vi "Caliper Setting UI_old.vi"(8 "error in (no error)":errorcluster, 11 "Vision_Image":T7(plugin-control)) -> (0 "error out":errorcluster, 2 "Cancel?":bool)   [LabVIEW 2015]
uses:
  Controls/CaliperType with Picture.ctl
  Controls/SelectionListEntry.ctl
  Controls/SelectionListEntryPointType.ctl
  Controls/CaliperDataEntry.ctl
  Controls/CaliperType.ctl
  Controls/CaliperResult.ctl
  Controls/Caliper_UI_Action_old.ctl
  Controls/AnalysisResultPointsAction.ctl
  Analysis/Controls/Analysis_Result_To_Caliper.ctl
panel:
  out "Result":string
  in  "DeleteCaliper":bool
  in  "CaliperList":i32(listbox)
  in  "AddCaliper":bool
  out "Result":T1
  out "CaliperEntryList":T2[](array[typedef]) {"CaliperType" items=["Distance", "Mid Point", "Perpendicular Projection", "Lines Intersection", "Angle from Horizontal", "Angle from Vertical", "Angle Defined by 3 Points", "Angle Defined by 4 Points", "Bissecting Line", "Mid Line", "Center of Mass", "Area", "Line Fit", "Circle Fit", "Ellipse Fit"]}
  out "AnalysisResultNum":i32
  out "SelectionList":T4[](array[typedef])
  out "Row":i32
  in  "Analysis Results":i32[](listbox) caption="Table"
  in  "CaliperType_w_Pic":T6 caption="Caliper Type" items=["Distance", "Mid Point", "Perpendicular Projection", "Lines Intersection", "Angle from Horizontal", "Angle from Vertical", "Angle Defined by 3 Points", "Angle Defined by 4 Points", "Bissecting Line", "Mid Line", "Center of Mass", "Area", "Line Fit", "Circle Fit", "Ellipse Fit"]
  in  "Cancel":bool
  in  "Done":bool
  in  "Run Algorithm":bool
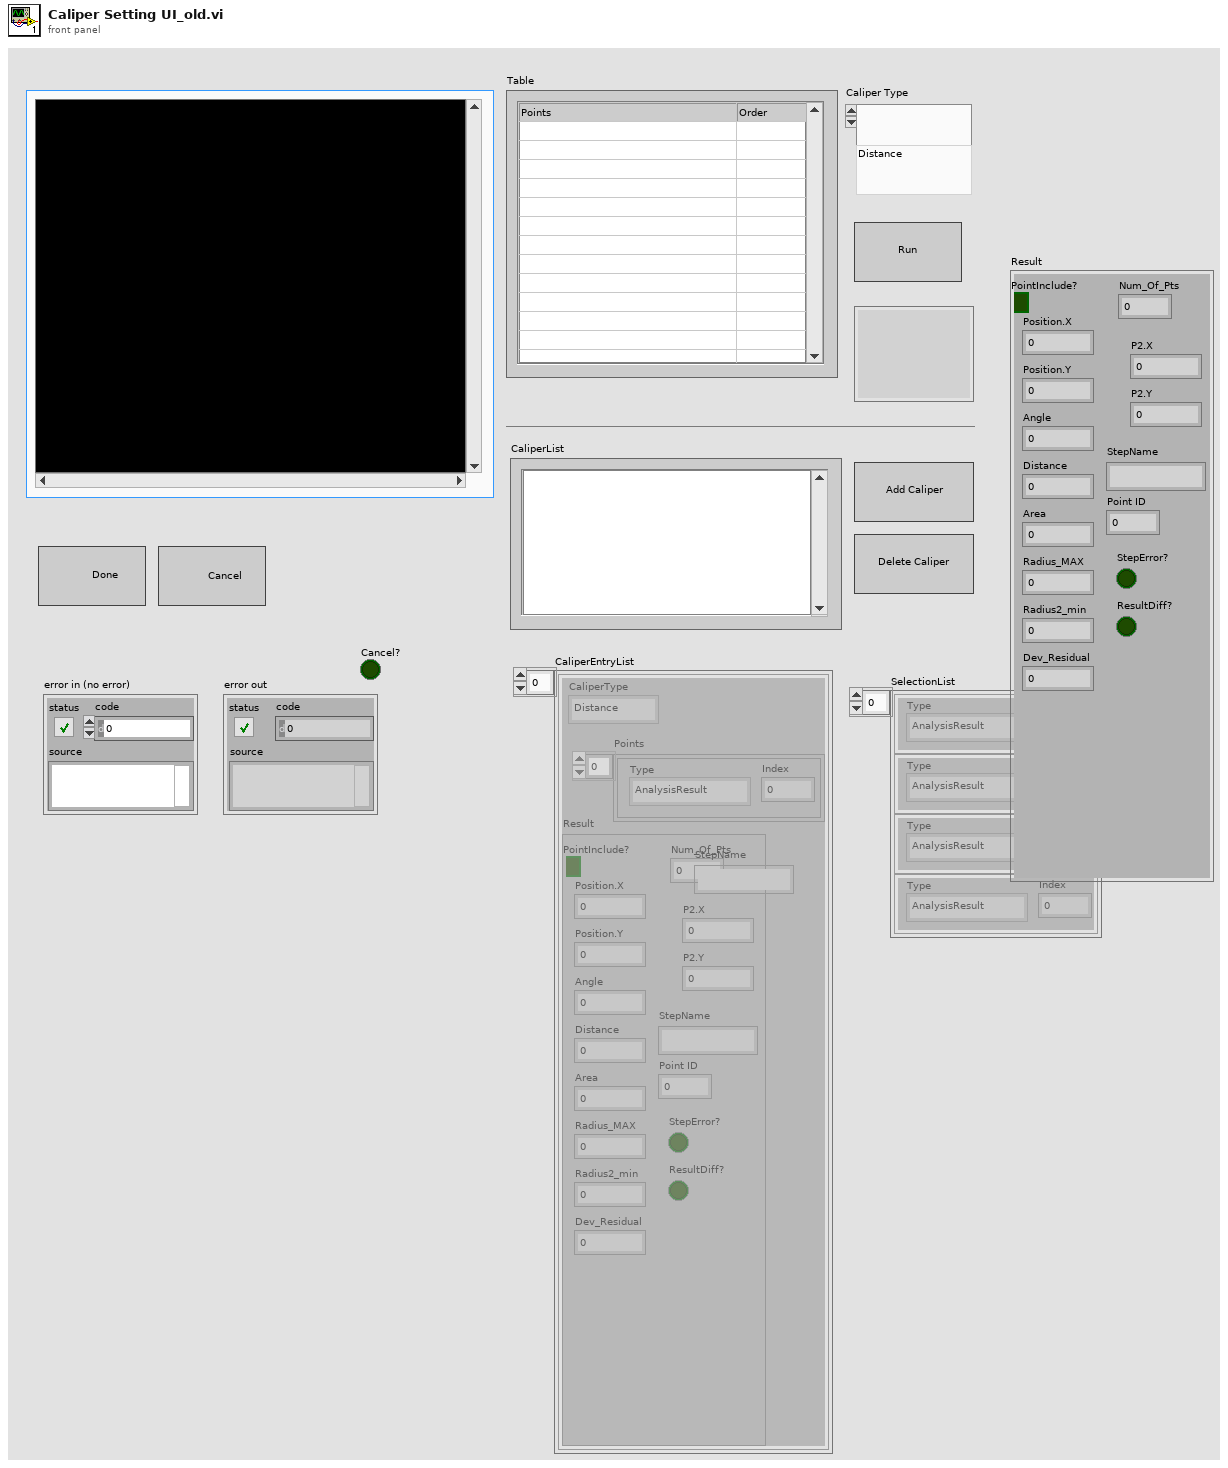
[diagram p1: front panel]
types:
  T1 = typedef "CaliperResult.ctl" = cluster{"PointInclude?":bool, "Num_Of_Pts":u8, "Position.X":dbl, "Position.Y":dbl, "Angle":dbl, "Distance":dbl, "Area":dbl, "Radius_MAX":dbl, "Radius2_min":dbl, "Dev_Residual":dbl, "P2.X":dbl, "P2.Y":dbl, "StepName":string, "Point ID":u8, "StepError?":bool, "ResultDiff?":bool}
  T2 = typedef "CaliperDataEntry.ctl" = cluster{"CaliperType":T3, "Points":T4[], "Result":T1, "StepName":string}
  T3 = typedef "CaliperType.ctl" = u32
  T4 = typedef "SelectionListEntry.ctl" = cluster{"Type":T5, "Index":i32}
  T5 = typedef "SelectionListEntryPointType.ctl" = enum16{"AnalysisResult", "CaliperResult"}
  T6 = typedef "CaliperType with Picture.ctl" = u32
  T7 = typedef "IMAQ Image.ctl" = refnum<image>
  T8 = typedef "Caliper_UI_Action_old.ctl" = enum16{"Init", "Done", "Cancel", "Run", "InitAnalysisResultTable", "UpdateSymbol", "UpdateOrderInTable", "UpdateAnalysisTable", "AddCaliperResultToTable", "AddCaliperEntry", "SetCaliperStepName", "UpdateCaliperList", "RemoveCaliperEntry", "ResetSelectionList"}
  T9 = typedef "Analysis_Result_To_Caliper.ctl" = cluster{"PointName":string, "Position_X":dbl, "Position_Y":dbl}
  T10 = typedef "AnalysisResultPointsAction.ctl" = enum16{"Init", "Add", "Delete", "ReplaceAll", "ReadAll", "Close"}
  T11 = typedef "CaliperDataEntry_SinglePoint.ctl" = cluster{"CaliperType":T3, "Points":T4[], "Result":T12, "StepName":string}
  T12 = typedef "CaliperResult_SinglePoint.ctl" = cluster{"PointInclude?":bool, "Position.X":dbl, "Position.Y":dbl, "Angle":dbl, "Distance":dbl, "Area":dbl, "Radius_MAX":dbl, "Radius2_min":dbl, "Dev_Residual":dbl, "StepName":string, "Point ID":u8, "StepError?":bool, "ResultDiff?":bool}
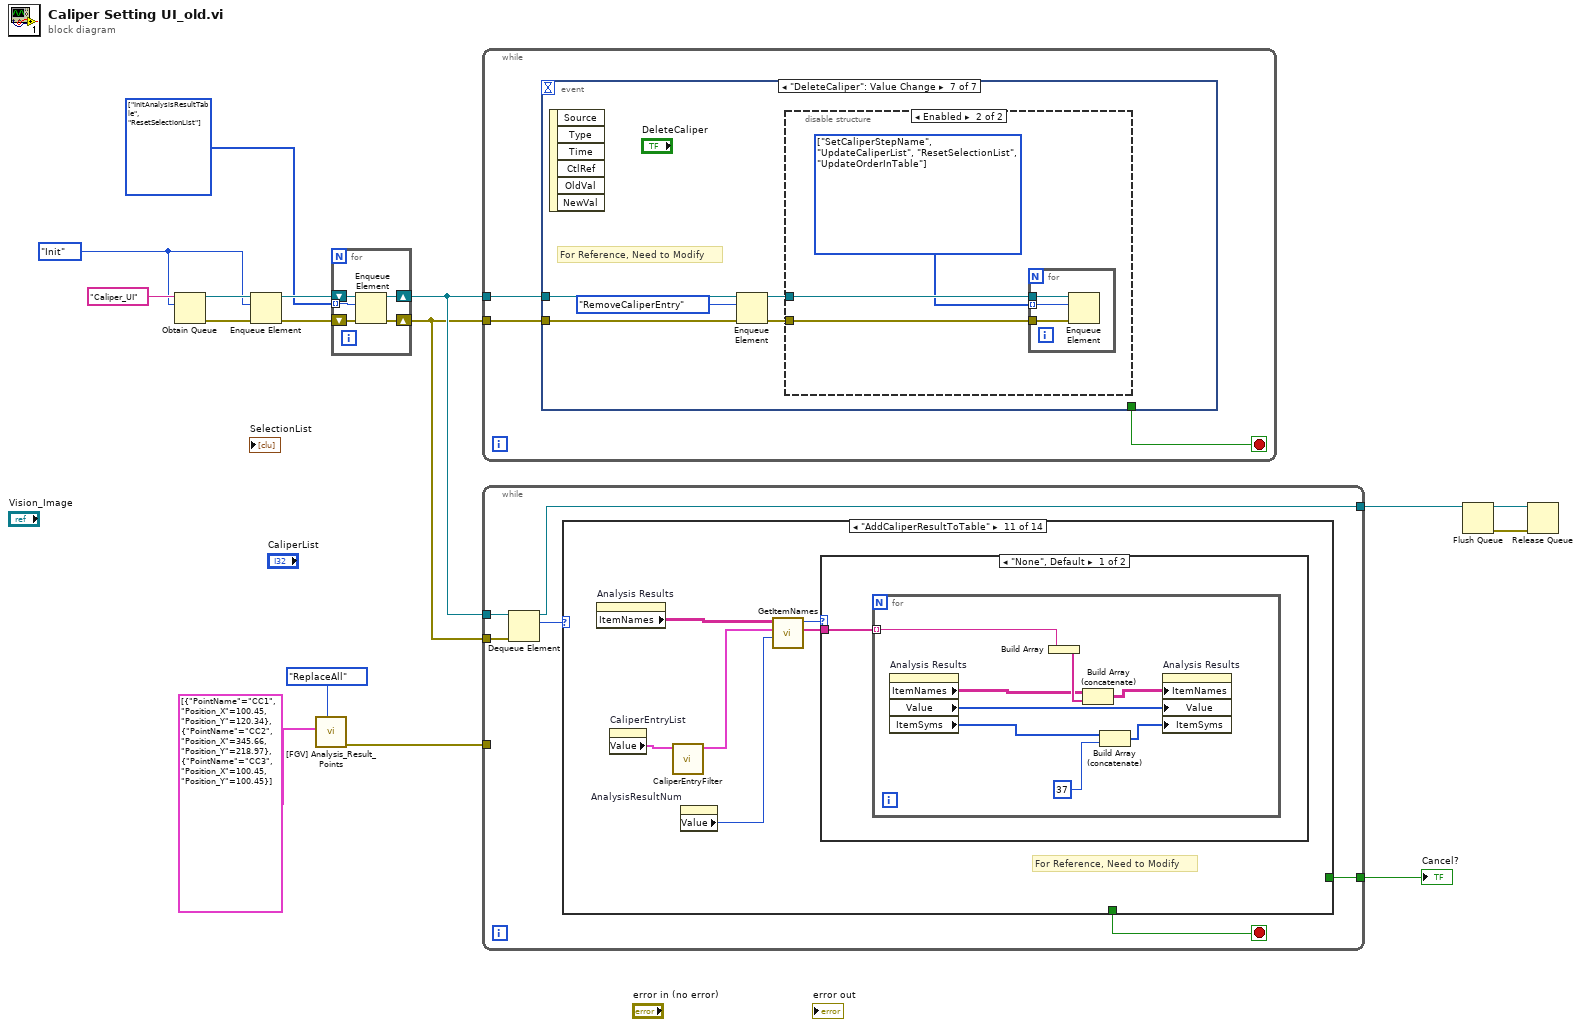
[diagram p0: block diagram]
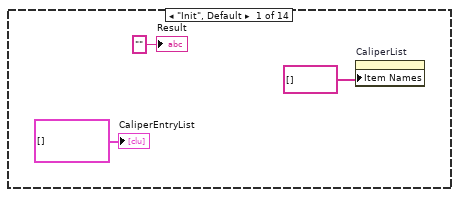
[diagram p2: hidden frame]
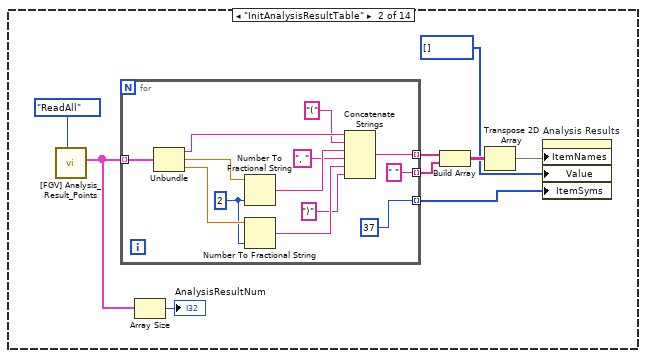
[diagram p3: hidden frame]
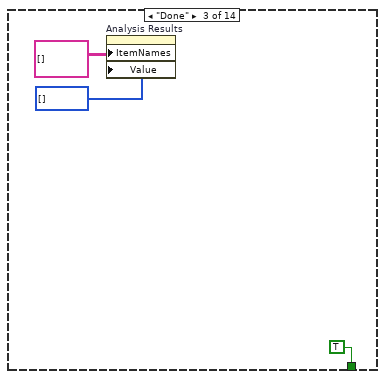
[diagram p4: hidden frame]
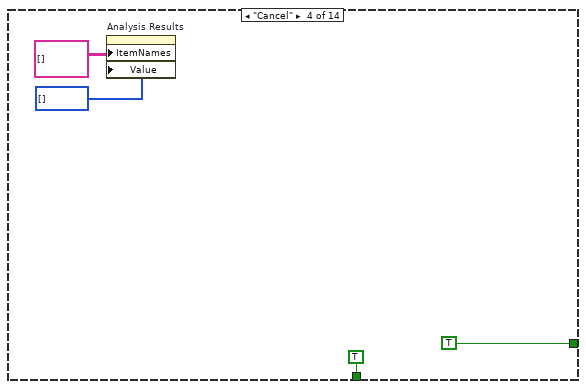
[diagram p5: hidden frame]
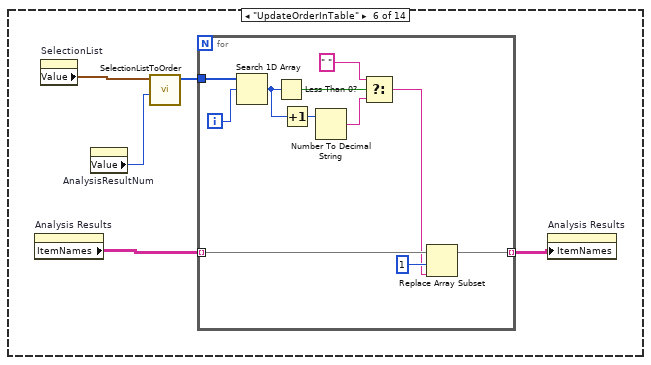
[diagram p7: hidden frame]
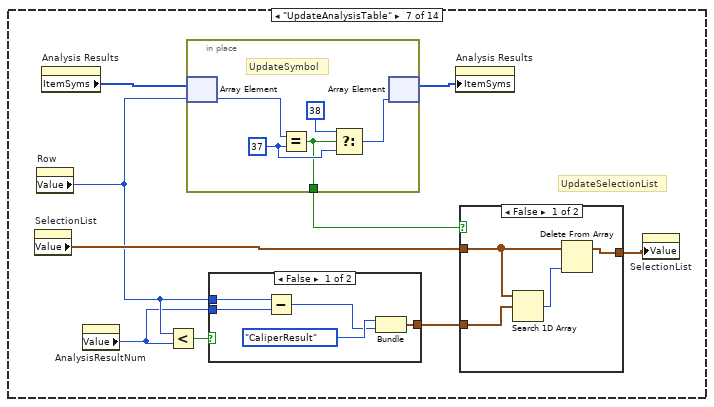
[diagram p8: hidden frame]
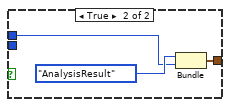
[diagram p9: hidden frame]
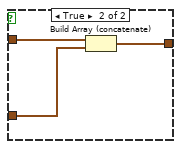
[diagram p10: hidden frame]
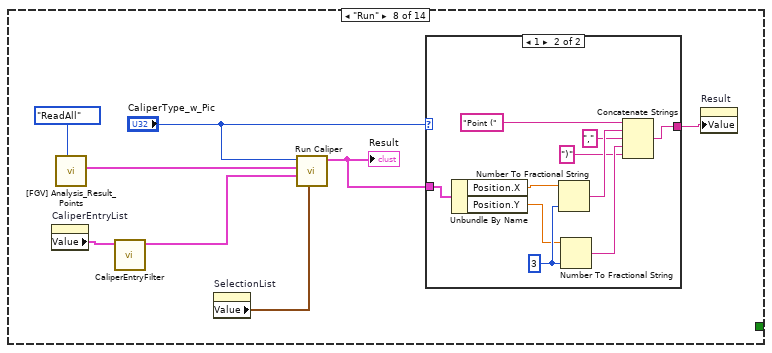
[diagram p11: hidden frame]
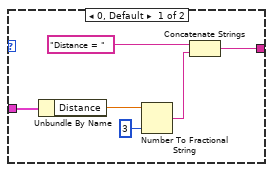
[diagram p12: hidden frame]
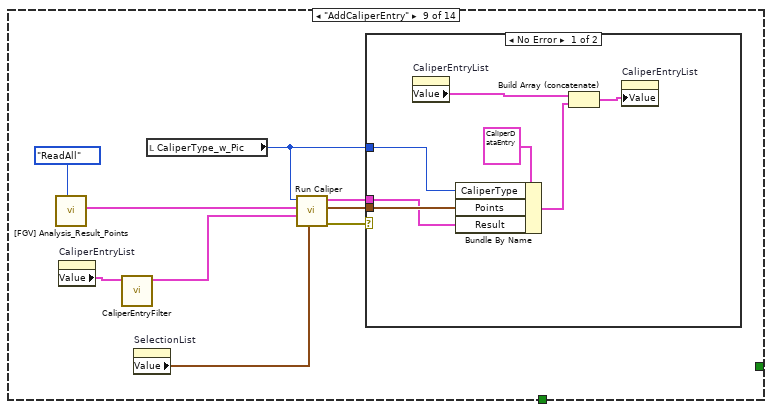
[diagram p13: hidden frame]
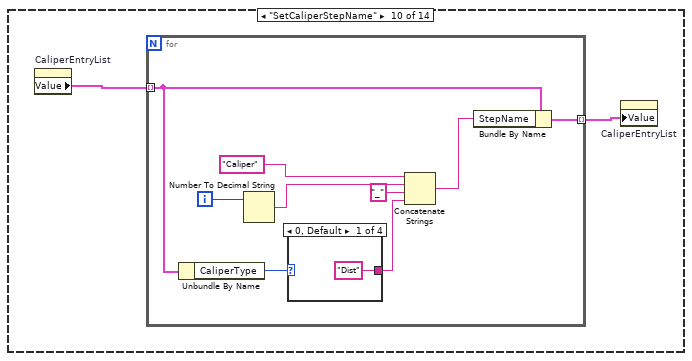
[diagram p15: hidden frame]
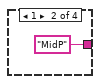
[diagram p16: hidden frame]
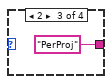
[diagram p17: hidden frame]
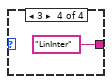
[diagram p18: hidden frame]
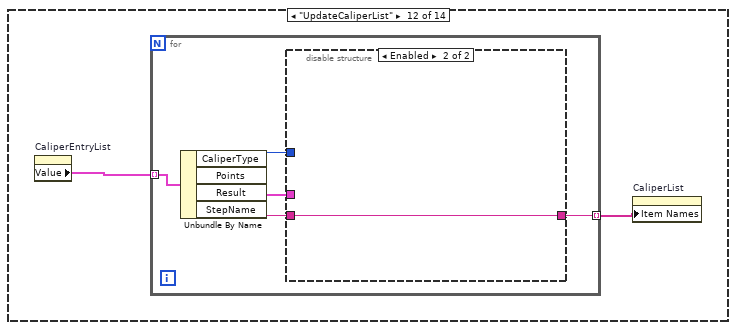
[diagram p20: hidden frame]
diagram:
  w1 = T8[] [enum."InitAnalysisResultTable", enum."ResetSelectionList"] items=["Init", "Done", "Cancel", "Run", "InitAnalysisResultTable", "UpdateSymbol", "UpdateOrderInTable", "UpdateAnalysisTable", "AddCaliperResultToTable", "AddCaliperEntry", "SetCaliperStepName", "UpdateCaliperList", "RemoveCaliperEntry", "ResetSelectionList"]
  w14 = Caliper_UI_Action_old."Init" ("CaliperAction")
  n1 = Obtain Queue(name (unnamed)="Caliper_UI", element data type=w14) -> (queue out=w15:refnum<queue>, error out=w9:errorcluster)  [unwired: 3 in, 1 out]
  n2 = Enqueue Element(queue=w15, element=w14, error in (no error)=w9) -> (queue out=w8:refnum<queue>, error out=w6:errorcluster)  [unwired: 1 in, 1 out]
  n3 = call "[FGV] Analysis_Result_Points.vi"("Action"=AnalysisResultPointsAction."ReplaceAll", "Analysis_Point_Result"=T9[] [{"PointName"="CC1", "Position_X"=100.45, "Position_Y"=120.34}, {"PointName"="CC2", "Position_X"=345.66, "Position_Y"=218.97}, {"PointName"="CC3", "Position_X"=100.45, "Position_Y"=100.45}]) -> ("error out"=w3:errorcluster)  [unwired: 8 in, 1 out]
  n4 = for {
    tunnel: w1 -> [w17] mode=indexing
    shift-right: [w20] -> w7
    shift-left: w8 -> [w21]
    shift-right: [w18] -> w5
    shift-left: w6 -> [w19]
    n5 = Enqueue Element(queue=w21, element=w17, error in (no error)=w19) -> (queue out=w20:refnum<queue>, error out=w18:errorcluster)  [unwired: 1 in, 1 out]
  }
  n6 = while {
    tunnel: w7 -> [w24]
    tunnel: w5 -> [w23]
    stop <- w22 stop-if-true
    n7 = event shown="[6] \"DeleteCaliper\": Value Change" {
      selector: _ -> [_ _ _ _ _ _ _]
      dyn-events: _ -> [_ _ _ _ _ _ _]
      timeout: _ -> [_ _ _ _ _ _ _]
      tunnel: w24 -> [_ w28 w32 w41 w45 w50 w67]
      tunnel: w23 -> [_ w27 w31 w40 w44 w49 w66]
      tunnel: [_ TRUE TRUE _ _ _ _] -> w22
      event Timeout {
        n8 = event-data() -> ()  [unwired: 1 in, 2 out]
      }
      event "Done": Value Change {
        n9 = event-data() -> ()  [unwired: 1 in, 6 out]
        n10 = Enqueue Element(queue=w28, element=Caliper_UI_Action_old."Done", error in (no error)=w27) -> ()  [unwired: 1 in, 3 out]
      }
      event "Cancel": Value Change {
        n11 = event-data() -> ()  [unwired: 1 in, 6 out]
        n12 = Enqueue Element(queue=w32, element=Caliper_UI_Action_old."Cancel", error in (no error)=w31) -> ()  [unwired: 1 in, 3 out]
      }
      event "Analysis Results": Double Click {
        n13 = event-data() -> ("Row"=→"Row":i32)  [unwired: 1 in, 8 out]
        n14 = Enqueue Element(queue=w41, element=Caliper_UI_Action_old."UpdateSymbol", error in (no error)=w40) -> (queue out=w38:refnum<queue>, error out=w37:errorcluster)  [unwired: 1 in, 1 out]
        n15 = Enqueue Element(queue=w38, element=Caliper_UI_Action_old."UpdateAnalysisTable", error in (no error)=w37) -> (queue out=w36:refnum<queue>, error out=w35:errorcluster)  [unwired: 1 in, 1 out]
        n16 = Enqueue Element(queue=w36, element=Caliper_UI_Action_old."UpdateOrderInTable", error in (no error)=w35) -> ()  [unwired: 1 in, 3 out]
      }
      event "Run Algorithm": Value Change {
        n17 = event-data() -> ()  [unwired: 1 in, 6 out]
        n18 = Enqueue Element(queue=w45, element=Caliper_UI_Action_old."Run", error in (no error)=w44) -> ()  [unwired: 1 in, 3 out]
      }
      event "AddCaliper": Value Change {
        # "For Reference, Need to Modify"
        n19 = event-data() -> ()  [unwired: 1 in, 6 out]
        n20 = Enqueue Element(queue=w50, element=Caliper_UI_Action_old."AddCaliperEntry", error in (no error)=w49) -> (queue out=w47:refnum<queue>, error out=w46:errorcluster)  [unwired: 1 in, 1 out]
        n21 = disable-structure shown="Enabled" {
          disable-tunnel: w47 -> [w55 w58]
          disable-tunnel: w46 -> [w53 w59]
          frame Disabled {
            n22 = Enqueue Element(queue=w55, element=Caliper_UI_Action_old."InitAnalysisResultTable", error in (no error)=w53) -> (queue out=w54:refnum<queue>, error out=w52:errorcluster)  [unwired: 1 in, 1 out]
            n23 = Enqueue Element(queue=w54, element=Caliper_UI_Action_old."AddCaliperResultToTable", error in (no error)=w52) -> ()  [unwired: 1 in, 3 out]
          }
          frame Enabled {
            w57 = T8[] [enum."SetCaliperStepName", enum."AddCaliperResultToTable", enum."UpdateCaliperList", enum."ResetSelectionList", enum."UpdateOrderInTable"] items=["Init", "Done", "Cancel", "Run", "InitAnalysisResultTable", "UpdateSymbol", "UpdateOrderInTable", "UpdateAnalysisTable", "AddCaliperResultToTable", "AddCaliperEntry", "SetCaliperStepName", "UpdateCaliperList", "RemoveCaliperEntry", "ResetSelectionList"]
            n24 = for {
              tunnel: w59 -> [w62]
              tunnel: w58 -> [w61]
              tunnel: w57 -> [w60] mode=indexing
              n25 = Enqueue Element(queue=w61, element=w60, error in (no error)=w62) -> ()  [unwired: 1 in, 3 out]
            }
          }
        }
      }
      event "DeleteCaliper": Value Change {
        # "For Reference, Need to Modify"
        n26 = event-data() -> ()  [unwired: 1 in, 6 out]
        n27 = Enqueue Element(queue=w67, element=Caliper_UI_Action_old."RemoveCaliperEntry", error in (no error)=w66) -> (queue out=w64:refnum<queue>, error out=w63:errorcluster)  [unwired: 1 in, 1 out]
        n28 = disable-structure shown="Enabled" {
          disable-tunnel: w64 -> [w72 w75]
          disable-tunnel: w63 -> [w70 w76]
          frame Disabled {
            n29 = Enqueue Element(queue=w72, element=Caliper_UI_Action_old."InitAnalysisResultTable", error in (no error)=w70) -> (queue out=w71:refnum<queue>, error out=w69:errorcluster)  [unwired: 1 in, 1 out]
            n30 = Enqueue Element(queue=w71, element=Caliper_UI_Action_old."AddCaliperResultToTable", error in (no error)=w69) -> ()  [unwired: 1 in, 3 out]
          }
          frame Enabled {
            w74 = T8[] [enum."SetCaliperStepName", enum."UpdateCaliperList", enum."ResetSelectionList", enum."UpdateOrderInTable"] items=["Init", "Done", "Cancel", "Run", "InitAnalysisResultTable", "UpdateSymbol", "UpdateOrderInTable", "UpdateAnalysisTable", "AddCaliperResultToTable", "AddCaliperEntry", "SetCaliperStepName", "UpdateCaliperList", "RemoveCaliperEntry", "ResetSelectionList"]
            n31 = for {
              tunnel: w76 -> [w79]
              tunnel: w75 -> [w78]
              tunnel: w74 -> [w77] mode=indexing
              n32 = Enqueue Element(queue=w78, element=w77, error in (no error)=w79) -> ()  [unwired: 1 in, 3 out]
            }
          }
        }
      }
    }
  }
  n33 = while {
    tunnel: w7 -> [w85]
    tunnel: w5 -> [w84]
    tunnel: [w82] -> w13
    tunnel: [w80] -> w10
    tunnel: w3 -> [_]
    stop <- w81 stop-if-true
    n34 = Dequeue Element(queue=w85, error in (no error)=w84) -> (queue out=w82:refnum<queue>, element=w83:T8)  [unwired: 1 in, 2 out]
    n35 = case shown="\"AddCaliperResultToTable\"" w83 {
      tunnel: [_ _ TRUE TRUE _ _ _ _ _ _ _ _ _ _] -> w81
      tunnel: [_ _ _ TRUE _ _ _ _ _ _ _ _ _ _] -> w80
      frame "Init", Default {
        n36 = property on="CaliperList" class="LstBox (strict)"("Item Names"=string[] []) -> ()  [unwired: 2 in, 2 out]
        "CaliperEntryList" <- T2[] [] ("CaliperEntryList")
        "Result" <- "" ("Result")
      }
      frame "InitAnalysisResultTable" {
        n37 = call "[FGV] Analysis_Result_Points.vi"("Action"=AnalysisResultPointsAction."ReadAll") -> ("Analysis_Point_Result Out"=w90:T9[])  [unwired: 9 in, 1 out]
        n38 = for {
          tunnel: w90 -> [w110] mode=indexing
          tunnel: [w100] -> w96 mode=indexing
          tunnel: [37] -> w95 mode=indexing
          tunnel: [" " ("string")] -> w91 mode=indexing
          w104 = i16 2 ("precision (6)")
          n39 = Unbundle(w110) -> ("PointName"=w107:string, "Position_X"=w109:dbl, "Position_Y"=w108:dbl)
          n40 = Number To Fractional String(number=w109, precision (6)=w104) -> (F-format string=w105:string)  [unwired: 2 in]
          n41 = Number To Fractional String(number=w108, precision (6)=w104) -> (F-format string=w102:string)  [unwired: 2 in]
          n42 = Concatenate Strings(w107, "(" ("string"), w105, ", " ("string"), w102, ")" ("string")) -> (w100:string)
        }
        n43 = Array Size(array=w90) -> (size(s)=→"AnalysisResultNum":i32)
        n44 = Build Array(w96, w91) -> (w94:string[][])
        n45 = Transpose 2D Array(2D array=w94) -> (transposed array=w92:string[][])
        n46 = property on="Analysis Results" class="MCListbox (strict)"("ItemNames"=w92, "Value"=i32[] [] ("Analysis Results"), "ItemSyms"=w95) -> ()  [unwired: 2 in, 2 out]
      }
      frame "Done" {
        n47 = property on="Analysis Results" class="MCListbox (strict)"("ItemNames"=string[][] [] ("Item Names"), "Value"=i32[] [] ("Analysis Results")) -> ()  [unwired: 2 in, 2 out]
      }
      frame "Cancel" {
        n48 = property on="Analysis Results" class="MCListbox (strict)"("ItemNames"=string[][] [] ("Item Names"), "Value"=i32[] [] ("Analysis Results")) -> ()  [unwired: 2 in, 2 out]
      }
      frame "UpdateSymbol" {
      }
      frame "UpdateOrderInTable" {
        n49 = property on="Analysis Results" class="MCListbox (strict)"() -> ("ItemNames"=w122:string[][])  [unwired: 2 in, 2 out]
        n50 = property on="SelectionList" class="Arr (strict)"() -> ("Value"=w120:T4[])  [unwired: 2 in, 2 out]
        n51 = property on="AnalysisResultNum" class="DigNum (strict)"() -> ("Value"=w119:i32)  [unwired: 2 in, 2 out]
        n52 = call "SelectionListToOrder.vi"("AnalysisResultNum"=w119, "SelectionList"=w120) -> ("Order"=w118:i32[])  [unwired: 9 in]
        n53 = for {
          tunnel: w118 -> [w133]
          tunnel: w122 -> [w131] mode=indexing
          tunnel: [w130] -> w121 mode=indexing
          i -> [w132]
          n54 = Search 1D Array(1D array=w133, element=w132) -> (index of element=w125:i32)  [unwired: 1 in]
          n55 = Less Than 0?(x=w125) -> (x < 0?=w128:bool)
          n56 = Increment(x=w125) -> (x+1=w123:i32)
          n57 = Number To Decimal String(number=w123) -> (decimal integer string=w124:string)  [unwired: 1 in]
          n58 = Select(t=" " ("new element/subarray"), s=w128, f=w124) -> (s? t:f=w126:string)
          n59 = Replace Array Subset(array=w131, new element=w126, index=1) -> (w130:string[])
        }
        n60 = property on="Analysis Results" class="MCListbox (strict)"("ItemNames"=w121) -> ()  [unwired: 2 in, 2 out]
      }
      frame "UpdateAnalysisTable" {
        # "UpdateSelectionList"
        n61 = property on="SelectionList" class="Arr (strict)"() -> ("Value"=w139:T4[])  [unwired: 2 in, 2 out]
        n62 = property on="Row" class="DigNum (strict)"() -> ("Value"=w136:i32)  [unwired: 2 in, 2 out]
        n63 = property on="Analysis Results" class="MCListbox (strict)"() -> ("ItemSyms"=w142:i32[])  [unwired: 2 in, 2 out]
        n64 = property on="AnalysisResultNum" class="DigNum (strict)"() -> ("Value"=w135:i32)  [unwired: 2 in, 2 out]
        n65 = Less?(x=w136, y=w135) -> (x < y?=w137:bool)
        n66 = in-place {
          in-place-border: [w158] -> w140
          w162 = 37 ("y")
          # "UpdateSymbol"
          n67 = in-place-array #1(w142, w136) -> (w160:i32)
          n68 = Equal?(x=w160, y=w162) -> (x = y?=w158:bool)
          n69 = Select(t=38 ("y"), s=w158, f=w162) -> (s? t:f=w159:i32)
          n70 = in-place-array #1(w159) -> (w141:i32[])  [unwired: 1 out]
        }
        n71 = case shown="False" w137 {
          tunnel: w136 -> [w145 w148]
          tunnel: [w146 w149] -> w134
          tunnel: w135 -> [w144 _]
          frame False {
            n72 = Subtract(x=w145, y=w144) -> (x-y=w143:i32)
            n73 = Bundle("Type"=SelectionListEntryPointType."CaliperResult", w143) -> (w146:cluster{"Type":T5, i32})  [unwired: 1 in]
          }
          frame True {
            n74 = Bundle("Type"=SelectionListEntryPointType."AnalysisResult", "Value"=w148) -> (w149:cluster{"Type":T5, "Value":i32})  [unwired: 1 in]
          }
        }
        n75 = property on="Analysis Results" class="MCListbox (strict)"("ItemSyms"=w141) -> ()  [unwired: 2 in, 2 out]
        n76 = case shown="False" w140 {
          tunnel: w139 -> [w154 w157]
          tunnel: [w153 w156] -> w138
          tunnel: w134 -> [w151 w155]
          frame False {
            n77 = Search 1D Array(1D array=w154, element=w151) -> (index of element=w152:i32)  [unwired: 1 in]
            n78 = Delete From Array(array=w154, index=w152) -> (array with subset deleted=w153:T4[])  [unwired: 1 in, 1 out]
          }
          frame True {
            n79 = Build Array (concatenate)(w157, w155) -> (w156:T4[])
          }
        }
        n80 = property on="SelectionList" class="Arr (strict)"("Value"=w138) -> ()  [unwired: 2 in, 2 out]
      }
      frame "Run" {
        n81 = property on="CaliperEntryList" class="Arr (strict)"() -> ("Value"=w167:T2[])  [unwired: 2 in, 2 out]
        n82 = call "[FGV] Analysis_Result_Points.vi"("Action"=AnalysisResultPointsAction."ReadAll") -> ("Analysis_Point_Result Out"=w169:T9[])  [unwired: 9 in, 1 out]
        n83 = call "CaliperEntryFilter.vi"("CaliperEntryList"=w167) -> ("FilteredCaliperEntry"=w166:T11[])  [unwired: 10 in]
        n84 = property on="SelectionList" class="Arr (strict)"() -> ("Value"=w168:T4[])  [unwired: 2 in, 2 out]
        n85 = call "Run Caliper.vi"("SelectionList"=w168, "FilteredCaliperEntry"=w166, "Analysis_Point_Result"=w169, "CaliperType"="CaliperType_w_Pic") -> ("Result"=w164:T1)  [unwired: 5 in, 2 out]
        "Result" <- w164
        n86 = case shown="1" "CaliperType_w_Pic" {
          tunnel: w164 -> [w176 w186]
          tunnel: [w171 w183] -> w163
          frame 0, Default {
            n87 = Unbundle By Name(w176) -> ("Distance"=w175:dbl)
            n88 = Number To Fractional String(number=w175, precision (6)=i16 3) -> (F-format string=w172:string)  [unwired: 2 in]
            n89 = Concatenate Strings("Distance = ", w172) -> (w171:string)
          }
          frame 1 {
            w182 = i16 3 ("precision (6)")
            n90 = Unbundle By Name(w186) -> ("Position.X"=w185:dbl, "Position.Y"=w181:dbl)
            n91 = Number To Fractional String(number=w185, precision (6)=w182) -> (F-format string=w180:string)  [unwired: 2 in]
            n92 = Number To Fractional String(number=w181, precision (6)=w182) -> (F-format string=w178:string)  [unwired: 2 in]
            n93 = Concatenate Strings("Point (", w180, "," ("string"), w178, ")" ("string")) -> (w183:string)
          }
        }
        n94 = property on="Result" class="Str"("Value"=w163) -> ()  [unwired: 2 in, 2 out]
      }
      frame "AddCaliperEntry" {
        n95 = call "[FGV] Analysis_Result_Points.vi"("Action"=AnalysisResultPointsAction."ReadAll") -> ("Analysis_Point_Result Out"=w194:T9[])  [unwired: 9 in, 1 out]
        n96 = property on="CaliperEntryList" class="Arr (strict)"() -> ("Value"=w188:T2[])  [unwired: 2 in, 2 out]
        n97 = call "CaliperEntryFilter.vi"("CaliperEntryList"=w188) -> ("FilteredCaliperEntry"=w187:T11[])  [unwired: 10 in]
        n98 = property on="SelectionList" class="Arr (strict)"() -> ("Value"=w193:T4[])  [unwired: 2 in, 2 out]
        n99 = local read "CaliperType_w_Pic"() -> (w189:T6)
        n100 = call "Run Caliper.vi"("SelectionList"=w193, "FilteredCaliperEntry"=w187, "Analysis_Point_Result"=w194, "CaliperType"=w189) -> ("error out"=w192:errorcluster, "SelectionListOut"=w190:T4[], "Result"=w191:T1)  [unwired: 5 in]
        n101 = case shown="No Error" w192 {
          tunnel: w191 -> [w197 _]
          tunnel: w190 -> [w198 _]
          tunnel: w189 -> [w199 _]
          frame No Error {
            n102 = property on="CaliperEntryList" class="Arr (strict)"() -> ("Value"=w202:T2[])  [unwired: 2 in, 2 out]
            n103 = Bundle By Name(cluster=T2 {"CaliperType"=0, "Points"=[], "Result"={"PointInclude?"=FALSE, "Num_Of_Pts"=0, "Position.X"=0.0, "Position.Y"=0.0, "Angle"=0.0, "Distance"=0.0, "Area"=0.0, "Radius_MAX"=0.0, "Radius2_min"=0.0, "Dev_Residual"=0.0, "P2.X"=0.0, "P2.Y"=0.0, "StepName"="", "Point ID"=0, "StepError?"=FALSE, "ResultDiff?"=FALSE}, "StepName"=""} ("CaliperEntry"), "CaliperType"=w199, "Points"=w198, "Result"=w197) -> (w196:T2)
            n104 = Build Array (concatenate)(w202, w196) -> (w201:T2[])
            n105 = property on="CaliperEntryList" class="Arr (strict)"("Value"=w201) -> ()  [unwired: 2 in, 2 out]
          }
          frame Error {
          }
        }
      }
      frame "SetCaliperStepName" {
        n106 = property on="CaliperEntryList" class="Arr (strict)"() -> ("Value"=w204:T2[])  [unwired: 2 in, 2 out]
        n107 = for {
          tunnel: w204 -> [w207] mode=indexing
          tunnel: [w205] -> w203 mode=indexing
          i -> [w212]
          n108 = Unbundle By Name(w207) -> ("CaliperType"=w213:T3)
          n109 = Number To Decimal String(number=w212) -> (decimal integer string=w210:string)  [unwired: 1 in]
          n110 = case shown="0, Default" w213 {
            tunnel: ["Dist" "MidP" "PerProj" "LinInter"] -> w208
            frame 0, Default {
            }
            frame 1 {
            }
            frame 2 {
            }
            frame 3 {
            }
          }
          n111 = Concatenate Strings("Caliper", w210, "_" ("string"), w208) -> (w206:string)
          n112 = Bundle By Name(cluster=w207, "StepName"=w206) -> (w205:T2)
        }
        n113 = property on="CaliperEntryList" class="Arr (strict)"("Value"=w203) -> ()  [unwired: 2 in, 2 out]
      }
      frame "AddCaliperResultToTable" {
        # "For Reference, Need to Modify"
        n114 = property on="Analysis Results" class="MCListbox (strict)"() -> ("ItemNames"=w222:string[][])  [unwired: 2 in, 2 out]
        n115 = property on="CaliperEntryList" class="Arr (strict)"() -> ("Value"=w223:T2[])  [unwired: 2 in, 2 out]
        n116 = call "CaliperEntryFilter.vi"("CaliperEntryList"=w223) -> ("FilteredCaliperEntry"=w221:T11[])  [unwired: 10 in]
        n117 = property on="AnalysisResultNum" class="DigNum (strict)"() -> ("Value"=w220:i32)  [unwired: 2 in, 2 out]
        n118 = call "GetItemNames.vi"("AnalysisResultNum"=w220, "FilteredCaliperEntry"=w221, "Item Names"=w222) -> ("NameTagToAdd"=w218:string[], "Action"=w219:enum16{"None", "Add", "Delete"})  [unwired: 7 in]
        n119 = case shown="\"None\", Default" w219 {
          tunnel: w218 -> [w224 _]
          frame "None", Default {
            n120 = for {
              tunnel: w224 -> [w225] mode=indexing
              n121 = property on="Analysis Results" class="MCListbox (strict)"() -> ("ItemNames"=w226:string[][], "Value"=w229:i32[], "ItemSyms"=w230:i32[])  [unwired: 2 in, 2 out]
              n122 = Build Array(w225) -> (w227:string[])
              n123 = Build Array (concatenate)(w226, w227) -> (w228:string[][])
              n124 = Build Array (concatenate)(w230, 37) -> (w232:i32[])
              n125 = property on="Analysis Results" class="MCListbox (strict)"("ItemNames"=w228, "Value"=w229, "ItemSyms"=w232) -> ()  [unwired: 2 in, 2 out]
            }
          }
          frame "Add" {
            # "No Need to Add More Points"
          }
        }
      }
      frame "UpdateCaliperList" {
        n126 = property on="CaliperEntryList" class="Arr (strict)"() -> ("Value"=w234:T2[])  [unwired: 2 in, 2 out]
        n127 = for {
          tunnel: w234 -> [w239] mode=indexing
          tunnel: [w235] -> w233 mode=indexing
          n128 = Unbundle By Name(w239) -> ("CaliperType"=w238:T3, "Result"=w237:T1, "StepName"=w236:string)  [unwired: 1 out]
          n129 = disable-structure shown="Enabled" {
            disable-tunnel: w238 -> [w242 _]
            disable-tunnel: w237 -> [w241 _]
            disable-tunnel: w236 -> [w240 w243]
            disable-tunnel: [_ w243] -> w235
            frame Disabled {
              n130 = case shown="0, Default" w242 {
                tunnel: w241 -> [_ _]
                tunnel: w240 -> [_ _]
                frame 0, Default {
                }
                frame 1 {
                }
              }
            }
            frame Enabled {
            }
          }
        }
        n131 = property on="CaliperList" class="LstBox (strict)"("Item Names"=w233) -> ()  [unwired: 2 in, 2 out]
      }
      frame "RemoveCaliperEntry" {
        n132 = property on="CaliperList" class="LstBox (strict)"() -> ("Value"=w245:i32)  [unwired: 2 in, 2 out]
        n133 = property on="CaliperEntryList" class="Arr (strict)"() -> ("Value"=w246:T2[])  [unwired: 2 in, 2 out]
        n134 = Delete From Array(array=w246, index=w245) -> (array with subset deleted=w244:T2[])  [unwired: 1 in, 1 out]
        n135 = property on="CaliperEntryList" class="Arr (strict)"("Value"=w244) -> ()  [unwired: 2 in, 2 out]
      }
      frame "ResetSelectionList" {
        n136 = property on="Analysis Results" class="MCListbox (strict)"() -> ("ItemSyms"=w247:i32[])  [unwired: 2 in, 2 out]
        n137 = for {
          tunnel: w247 -> [_] mode=indexing
          tunnel: [37 ("y")] -> w248 mode=indexing
        }
        n138 = property on="Analysis Results" class="MCListbox (strict)"("ItemSyms"=w248) -> ()  [unwired: 2 in, 2 out]
        n139 = property on="SelectionList" class="Arr (strict)"("Value"=T4[] [] ("SelectionList")) -> ()  [unwired: 2 in, 2 out]
      }
    }
  }
  "Cancel?" <- w10
  n140 = Flush Queue(queue=w13) -> (queue out=w12:refnum<queue>, error out=w11:errorcluster)  [unwired: 1 in, 1 out]
  n141 = Release Queue(queue=w12, error in (no error)=w11) -> ()  [unwired: 1 in, 3 out]
